vi "getEMGain.vi"(6 "Delay between send and receive [ms]":i32=100, 8 "error in (no error)":errorcluster, 11 "CCD in":refnum<class "CCD.lvclass">) -> (0 "error out":errorcluster, 2 "gain":i32, 3 "CCD out":refnum<class "CCD.lvclass">)   [LabVIEW 2020, in "horiba.lvlib" / "CCD.lvclass"]
doc: "Gets the current gain token and the associated description information for the gain token. Gain tokens and their descriptions are part of the CCD configuration information. See ccd_getConfig command.\nFor example:\n\n\"gains\": [\n {\n \"info\": \"Best Dynamic Range\",\n \"token\": 1\n },\n {\n \"info\": \"High Sensitivity\",\n \"token\": 2\n },\n {\n \"info\": \"High Light\",\n \"token\": 0\n }\n]"
uses:
  CCD.lvclass
  CCD.lvclass/CCD.ctl
  20f7d3bd-08ac-4524-9bed-df36c1da25a0.vi
  a21955fc-e3a0-4e36-8495-41f1bfac7860.vi
  GenericDevice/GenericDevice.lvclass
  EMGain.ctl
panel:
  # "Connector Pane"
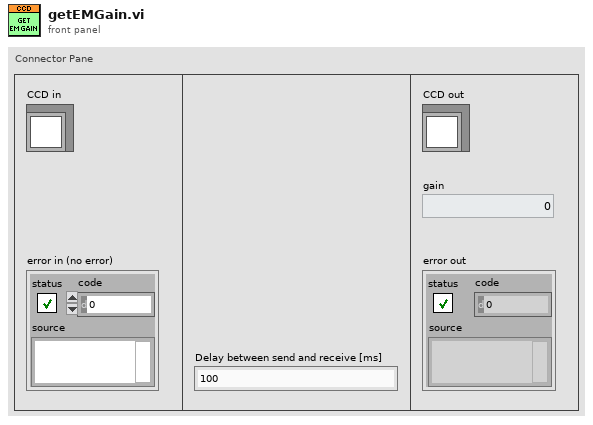
[diagram p1: front panel]
types:
  T1 = typedef "horiba.lvlib/CCD.lvclass/EMGain.ctl" = cluster{"gain":i32}
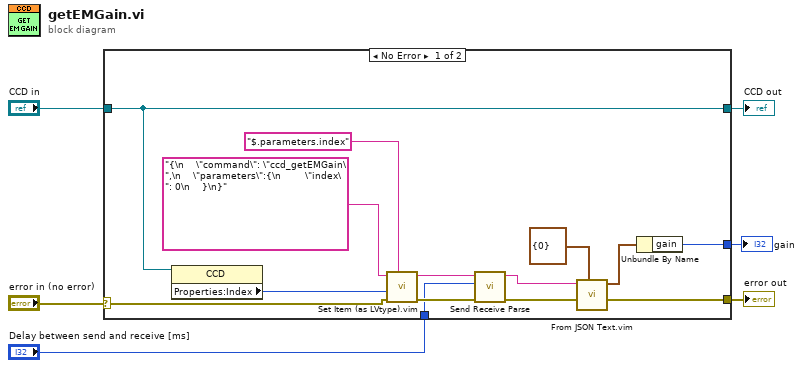
[diagram p0: block diagram]
diagram:
  n1 = case shown="No Error" "error in (no error)" {
    selector: "error in (no error)" -> [w16 w22]
    tunnel: [w15 w22] -> w5
    tunnel: [w18 w21] -> w3
    tunnel: "CCD in" -> [w18 w21]
    tunnel: [w10 _] -> w1
    tunnel: "Delay between send and receive [ms]" -> [w9 _]
    frame No Error {
      n2 = property on="Property Node" class="CCD"(reference=w18) -> ("Properties:Index"=w17:i32)  [unwired: 1 in, 2 out]
      n3 = call "Set Item (as LVtype).vim"("$Path or Item Name"="$.parameters.index", "error in (no error)"=w16, "Anything"=w17, "JSON"="{\n    \"command\": \"ccd_getEMGain\",\n    \"parameters\":{\n        \"index\": 0\n    }\n}") -> ("error out"=w12:errorcluster, "<JSON>"=w8:string)  [unwired: 4 in, 1 out]
      n4 = call "Send Receive Parse.vi"("error in"=w12, "Delay between send and receive [ms]"=w9, "<JSON>"=w8) -> ("error out"=w13:errorcluster, "results-JSON string"=w14:string)  [unwired: 6 in, 1 out]
      n5 = call "From JSON Text.vim"("Data Type and Default Value"=T1 {"gain"=0} ("gain"), "error in (no error)"=w13, "JSON"=w14) -> ("error out"=w15:errorcluster, "Data out"=w11:T1)  [unwired: 7 in]
      n6 = Unbundle By Name(w11) -> ("gain"=w10:i32)
    }
    frame Error {
    }
  }
  "error out" <- w5
  "CCD out" <- w3
  "gain" <- w1
